vi "PythonHandlerNodeTest.vi"() -> ()   [LabVIEW 2014]
uses:
  <vilib>/event_ctls.llb/lveventtype.ctl
panel:
  out "Array":string[](array[string])
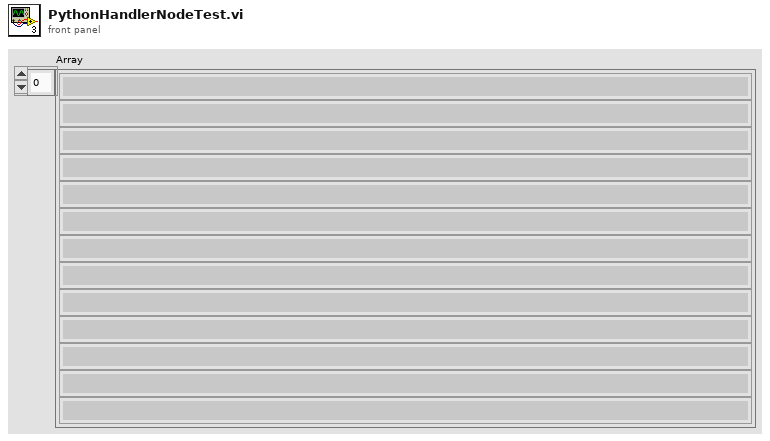
[diagram p1: front panel]
types:
  T1 = typedef "lveventtype.ctl" = enum32{"Null", "Timeout", "Annotation Menu Selection", "Annotation Menu Selection?", "App Instance Close", "App Instance Close?", "Autoscale Range Change", "Bookmark Info Change", "Cell Edit", "Cell Edit?", "Cursor Grab", "Cursor Grab?", "Cursor Menu Selection", "Cursor Menu Selection?", "Cursor Move", "Cursor Release", "Data Change", "Direction Change", "Display State Change", "Drag Ended", "Drag Enter", "Drag Leave", "Drag Over", "Drag Source Update", "Drag Starting", "Drag Starting?", "Drop", "Exec State Change", "Key Down", "Key Down?", "Key Repeat", "Key Repeat?", "Key Up", "Listbox Double Click", "Menu Activation?", "Menu Selection (App)", "Menu Selection? (App)", "Menu Selection (User)", "Mouse Down", "Mouse Down?", "Mouse Enter", "Mouse Leave", "Mouse Move", "Mouse Up", "Mouse Wheel", "NI Security User Change (App)", "Pane Size", "Panel Close", "Panel Close?", "Panel Resize", "Plot Attribute Change", "Scale Range Change", "Shortcut Menu Activation?", "Shortcut Menu Selection (App)", "Shortcut Menu Selection? (App)", "Shortcut Menu Selection (User)", "Tree Double Click", "Tree Drag", "Tree Drag?", "Tree Drop", "Tree Drop?", "Tree Item Close", "Tree Item Close?", "Tree Item Open", "Tree Item Open?", "User Event", "Value Change"}
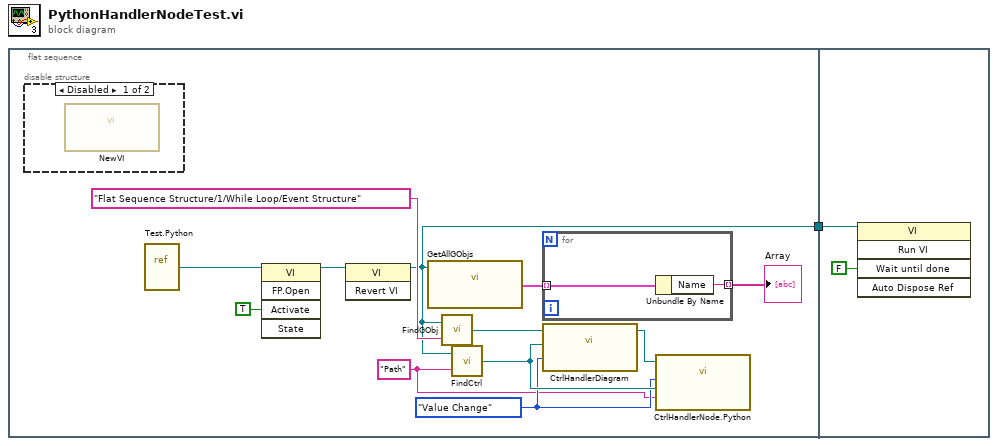
[diagram p0: block diagram]
diagram:
  n1 = flat-sequence {
    tunnel: [w5] -> w1
    tunnel: w1 -> [w16]
    frame #0 {
      w7 = lveventtype."Value Change" ("Type")
      w6 = "Path" ("Name")
      n2 = disable-structure shown="Disabled" {
        frame Disabled {
          n3 = call "NewVI.vi"() -> ()  [unwired: 3 in, 1 out]
        }
        frame Enabled {
        }
      }
      n4 = vi-ref "Test.Python.vi"() -> (w3:refnum<vi>)
      n5 = invoke class="VI" method="FP.Open"(reference=w3, "Activate"=TRUE ("Activate?")) -> (reference out=w2:refnum<vi>)  [unwired: 3 in, 4 out]
      n6 = invoke class="VI" method="Revert VI"(reference=w2) -> (reference out=w5:refnum<vi>)  [unwired: 2 in, 2 out]
      n7 = call "GetAllGObjs.vi"("VI"=w5) -> ("GObjs"=w13:cluster{"Name":string, "GObj":refnum<vi>}[])  [unwired: 1 in]
      n8 = call "FindGObj.vi"("Name"="Flat Sequence Structure/1/While Loop/Event Structure", "VI"=w5) -> ("GObj"=w10:refnum<vi>)
      n9 = call "FindCtrl.vi"("Name"=w6, "VI"=w5) -> ("Ctrl"=w8:refnum<vi>)
      n10 = for {
        tunnel: w13 -> [w15] mode=indexing
        tunnel: [w14] -> w12 mode=indexing
        n11 = Unbundle By Name(w15) -> ("Name"=w14:string)
      }
      "Array" <- w12
      n12 = call "CtrlHandlerDiagram.vi"("Type"=w7, "Ctrl"=w8, "Structure"=w10) -> ("Diagram"=w9:refnum<vi>)  [unwired: 1 out]
      n13 = call "CtrlHandlerNode.Python.vi"("Diagram"=w9, "Name"=w6, "Ctrl"=w8, "Type"=w7) -> ()  [unwired: 1 in]
    }
    frame #1 {
      n14 = invoke class="VI" method="Run VI"(reference=w16, "Wait until done"=FALSE ("Wait Until Done")) -> ()  [unwired: 3 in, 5 out]
    }
  }
